vi "Extract3ColumnsDisplay.vi"(8 "Error In":errorcluster, 11 "Input Array":string[][](array[string])) -> (0 "Error Out":errorcluster, 2 "appended array":string[][](array[string]), 3 "Array of filtered rows":string[][][](array[string]))   [LabVIEW 2014]
uses:
  Tables/scan_array.llb/Scan Array (I32).vi
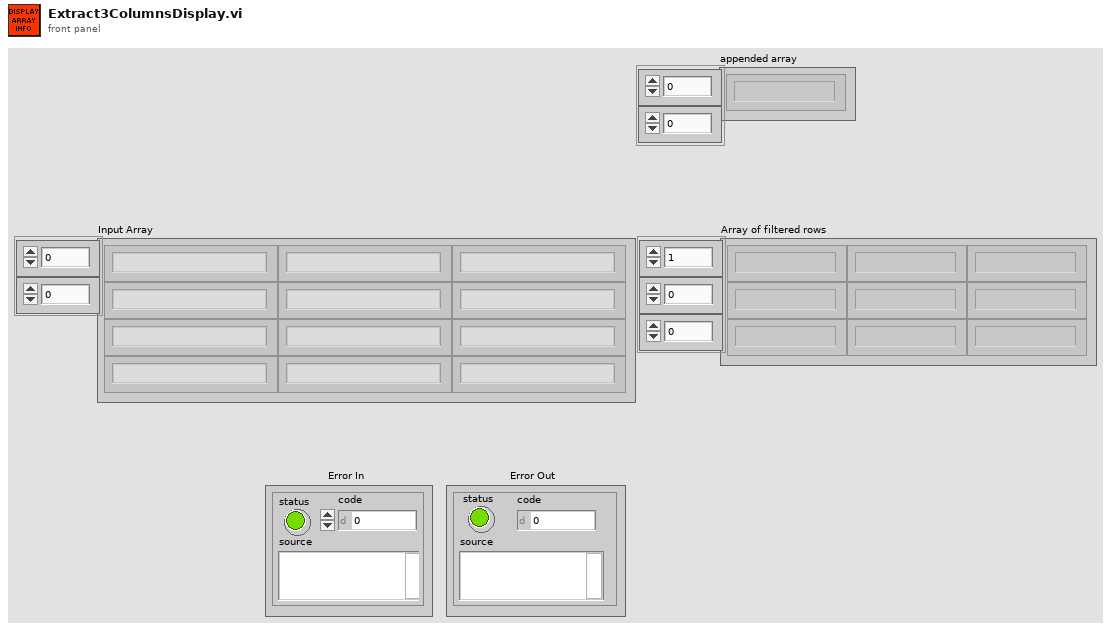
[diagram p1: front panel]
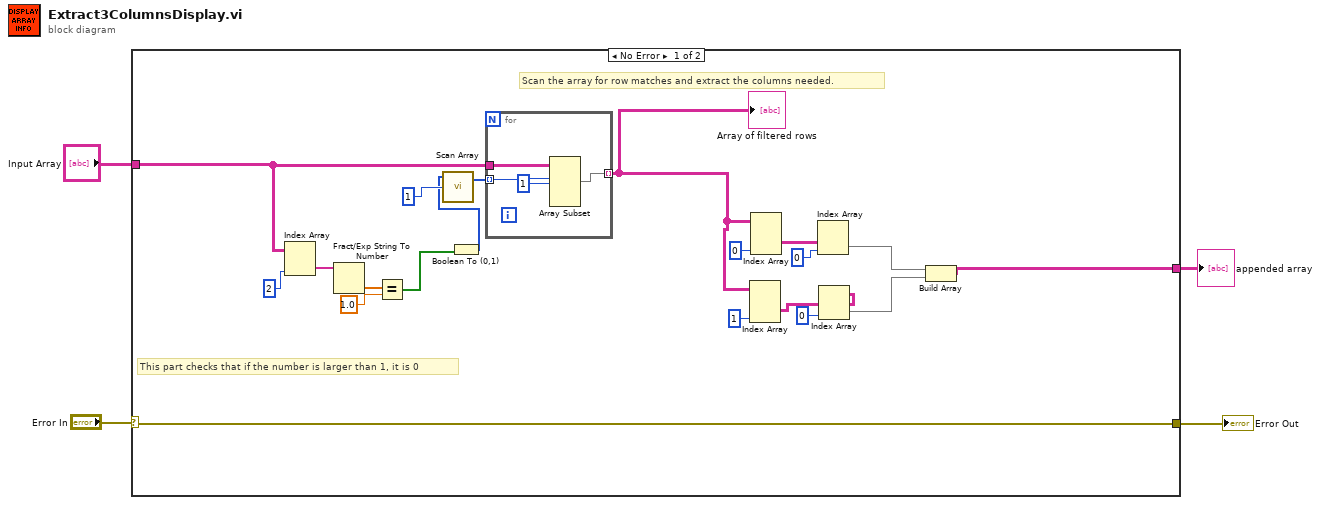
[diagram p0: block diagram]
diagram:
  n1 = case shown="No Error" "Error In" {
    selector: "Error In" -> [w5 w29]
    tunnel: [w5 w29] -> w4
    tunnel: "Input Array" -> [w7 _]
    tunnel: [w6 _] -> w2
    frame No Error {
      # "This part checks that if the number is larger than 1, it is 0"
      # "Scan the array for row matches and extract the columns needed."
      n2 = Index Array(array=w7, index (col)=2 ("disabled index (col)")) -> (element=w21:string[])  [unwired: 1 in]
      n3 = Fract/Exp String To Number(string=w21) -> (number=w19:dbl[])  [unwired: 3 in, 1 out]
      n4 = Equal?(x=w19, y=1.0) -> (x = y?=w17:bool[])
      n5 = Boolean To (0,1)(Boolean=w17) -> (0, 1=w18:i16[])
      n6 = call-poly "Scan Array.vi"("search element"=1, "Input array"=w18) -> ("Matched Indices"=w24:i32[])  [unwired: 3 in]
      n7 = for {
        tunnel: w24 -> [w28] mode=indexing
        tunnel: [w26] -> w14 mode=indexing
        tunnel: w7 -> [w25]
        n8 = Array Subset(array=w25, index (row)=w28, length (row)=1 ("length")) -> (w26:string[][])  [unwired: 2 in]
      }
      "Array of filtered rows" <- w14
      n9 = Index Array(array=w14, index (dim 2)=1 ("index (col)")) -> (element=w13:string[][])  [unwired: 2 in]
      n10 = Index Array(array=w14, index (dim 2)=0 ("disabled index (col)")) -> (element=w12:string[][])  [unwired: 2 in]
      n11 = Index Array(array=w12, index (col)=0 ("disabled index (col)")) -> (element=w8:string[])  [unwired: 1 in]
      n12 = Index Array(array=w13, index (col)=0 ("disabled index (col)")) -> (element=w9:string[])  [unwired: 1 in]
      n13 = Build Array(w8, w9) -> (w6:string[][])
    }
    frame Error {
    }
  }
  "Error Out" <- w4
  "appended array" <- w2
